vi "WaveformAcquisitionSynchronous (subVI).vi"(4 "Handle":i32, 5 "ADC Rate (ms)":dbl=1.0 min=0.033333 max=5.0 format="%.4f", 6 "Number of Positions to Read":u32=2 min=2 max=10000, 7 "Data Array In":dbl[](array[numeric]) format="%.2f", 8 "DAC Rate (ms)":dbl=1.0 min=0.0333333 max=5.0 format="%.4f", 9 "Number of Steps":u32=2 min=1 max=1000, 10 "Axis":u32) -> (2 "Data Array Out":dbl[](array[numeric]) format="%.2f", 3 "Return Code":i32)   [LabVIEW 2012]
uses:
  Madlib.dll
panel:
  # "This example demonstrates the two step process of simultaneous triggering a waveform read/write on a single axis."
  # "X = 1\nY = 2\nZ = 3"
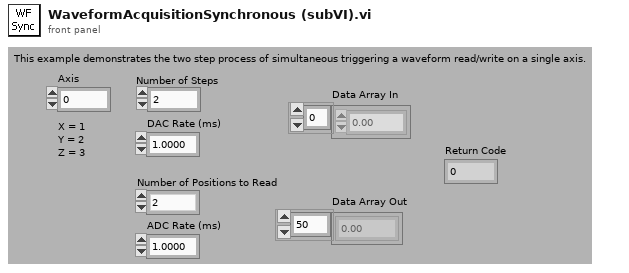
[diagram p1: front panel]
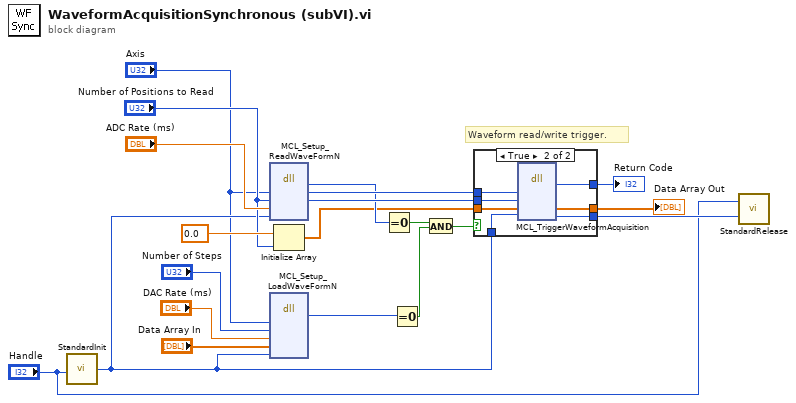
[diagram p0: block diagram]
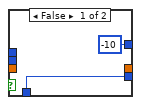
[diagram p2: hidden frame]
diagram:
  # "Waveform read/write trigger."
  n1 = call "StandardInit.vi"("Incoming Handle"="Handle") -> ("Outgoing Handle"=w7:i32)
  n2 = dll-call lib="C:/Users/Labview/Desktop/SRR/Madlib_x64/Labview Examples/MADLib.dll" fn="MCL_Setup_ReadWaveFormN" label="Setup WF Read"("axis"="Axis", "DataPoints"="Number of Positions to Read", "milliseconds"="ADC Rate (ms)", "handle"=w7) -> (w15:i32, "axis"=w18:u32, "DataPoints"=w17:u32)  [unwired: 5 in, 2 out]
  n3 = dll-call lib="C:/Users/Labview/Desktop/SRR/Madlib_x64/Labview Examples/MADLib.dll" fn="MCL_Setup_LoadWaveFormN" label="Setup WF Load"("axis"="Axis", "DataPoints"="Number of Steps", "milliseconds"="DAC Rate (ms)", "waveform"="Data Array In", "handle"=w7) -> (w14:i32)  [unwired: 8 in, 2 out]
  n4 = Initialize Array(0.0, "Number of Positions to Read") -> (w10:dbl[])
  n5 = Equal To 0?(x=w15) -> (x = 0?=w20:bool)
  n6 = Equal To 0?(x=w14) -> (x = 0?=w19:bool)
  n7 = And(x=w20, y=w19) -> (x .and. y?=w16:bool)
  n8 = case shown="True" w16 {
    tunnel: [_ w29] -> w2
    tunnel: w18 -> [_ w28]
    tunnel: w17 -> [_ w27]
    tunnel: w10 -> [_ w26]
    tunnel: w7 -> [w22 w25]
    tunnel: [w22 w24] -> w6
    tunnel: [-10 w23] -> w3
    frame False {
    }
    frame True {
      n9 = dll-call lib="C:/Users/Labview/Desktop/SRR/Madlib_x64/Labview Examples/MADLib.dll" fn="MCL_TriggerWaveformAcquisition"("axis"=w28, "DataPoints"=w27, "waveform"=w26, "handle"=w25) -> (w23:i32, "waveform"=w29:dbl[], "handle"=w24:i32)  [unwired: 5 in, 2 out]
    }
  }
  "Data Array Out" <- w2
  "Return Code" <- w3
  n10 = call "StandardRelease.vi"("Outgoing Handle"=w6, "Incoming Handle"="Handle") -> ()  [unwired: 1 in]
